vi "visualizer globals.vi"() -> ()   [LabVIEW 2016, in "FPGA RM System Definition API.lvlib"]
uses:
  FPGA RM System Definition API.lvlib
panel:
  in  "Datatype Filter":string
  in  "Input Type Filter":string
  in  "Resource Name Filter":string
  in  "RIO Device Name Filter":string
  in  "selected columns":bool[](array[boolean])=[TRUE, TRUE, TRUE, TRUE, TRUE, TRUE]
  in  "show unmapped?":bool=TRUE
  in  "show mapped?":bool=TRUE
  in  "Sort Types":string[](array[string])=["FPGA CD", "resource", "input type", "datatype", "reserver", "notes"]
  in  "Visualizer Status":string="rm.visualizer.status"
  in  "viz.sidebar.min":i32=30
  in  "viz.sidebar.max":i32=270
  in  "character size":i32=7
  in  "max column width":i32=400
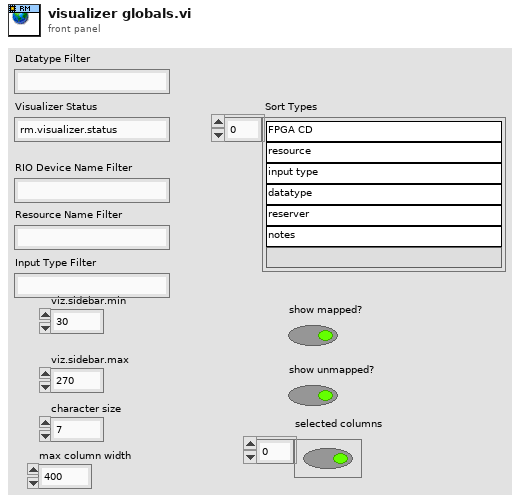
[diagram p1: front panel]
diagram:
